vi "Bubble Sort Person Array Using Functors.vi"(9 "Swapper":refnum<class "Swapper.lvclass">, 11 "Unsorted":T1[](array[typedef]) {"Birth Date" format="%<%Y/%b/%d>T"}) -> (3 "Sorted":T1[](array[typedef]) {"Birth Date" format="%<%Y/%b/%d>T"})   [LabVIEW 2023]
doc: "This VI implements a basic Bubble Sort for the array data, using the provided VI reference as the comparison function for two elements."
uses:
  Swapper/Swapper.lvclass
  Person Information.ctl
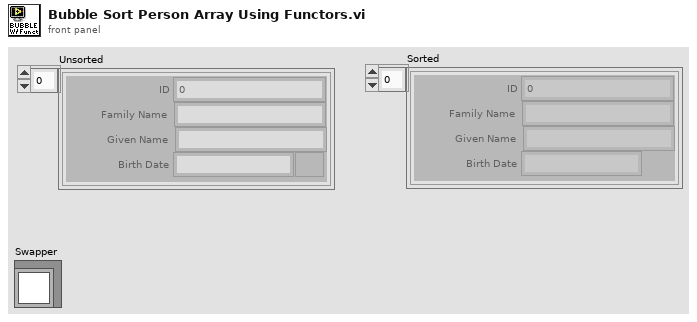
[diagram p1: front panel]
types:
  T1 = typedef "Person Information.ctl" = cluster{"ID":u32, "Family Name":string, "Given Name":string, "Birth Date":timestamp}
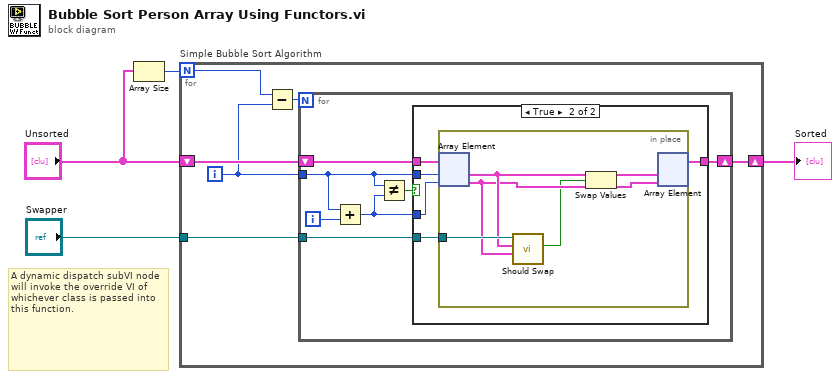
[diagram p0: block diagram]
diagram:
  # "A dynamic dispatch subVI node will invoke the override VI of whichever class is passed into this function."
  n1 = Array Size(array="Unsorted") -> (size(s)=w4:i32)
  n2 = for "Simple Bubble Sort Algorithm" {
    N: w4 -> [w7]
    shift-right: [w9] -> w3
    shift-left: "Unsorted" -> [w10]
    tunnel: "Swapper" -> [w6]
    i -> [w5]
    n3 = Subtract(x=w7, y=w5) -> (x-y=w8:i32)
    n4 = for {
      N: w8 -> [_]
      shift-right: [w16] -> w9
      shift-left: w10 -> [w17]
      tunnel: w5 -> [w12]
      tunnel: w6 -> [w11]
      i -> [w14]
      n5 = Add(x=w12, y=w14) -> (x+y=w13:i32)
      n6 = Not Equal?(x=w12, y=w13) -> (x != y?=w15:bool)
      n7 = case shown="True" w15 {
        tunnel: w17 -> [w18 w23]
        tunnel: [w18 w22] -> w16
        tunnel: w12 -> [_ w21]
        tunnel: w13 -> [_ w20]
        tunnel: w11 -> [_ w19]
        frame False {
        }
        frame True {
          n8 = in-place {
            in-place-border: w19 -> [w27]
            n9 = in-place-array #1(w23, w21, w20) -> (w26:T1, w25:T1)
            n10 = call-dynamic "Should Swap.vi"("Person B"=w25, "Person A"=w26, "Swapper in"=w27) -> ("Swap?"=w24:bool)  [unwired: 8 in]
            n11 = Swap Values(12:w26, 13:w24, 14:w25) -> (1:w29:T1, 3:w28:T1)
            n12 = in-place-array #1(w29, w28) -> (w22:T1[])  [unwired: 2 out]
          }
        }
      }
    }
  }
  "Sorted" <- w3
